vi "Release Queue.vi"(8 "error in (no error)":errorcluster, 11 "LVQueue Sink in":refnum<class "LVQueue Sink.lvclass">) -> (0 "error out":errorcluster, 3 "Remaining Elements":T1[](array[typedef]))   [LabVIEW 2018, in "MVA Framework.lvlib" / "LVQueue Sink.lvclass"]
uses:
  LVQueue Sink.lvclass
  Composed Log/Types/Log Level.ctl
  Composed Log/Composed Log.lvlib
  Composed Log/Types/Log Packet.ctl
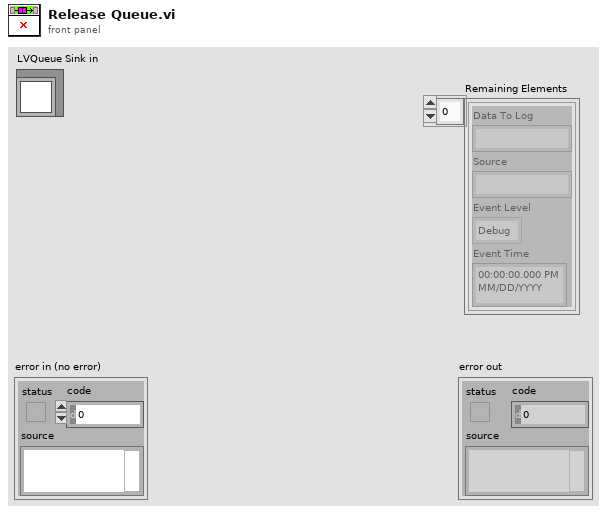
[diagram p1: front panel]
types:
  T1 = typedef "MVA Framework.lvlib/Composed Log.lvlib/Log Packet.ctl" = cluster{"Data To Log":string, "Source":string, "Event Level":T2, "Event Time":timestamp}
  T2 = typedef "MVA Framework.lvlib/Composed Log.lvlib/Log Level.ctl" = enum16{"Debug", "Info", "Warning", "Error", "Critical"}
  T3 = typedef "Composed Log.lvlib/Application Logger.lvclass/Log Packet.ctl" = cluster{"Data To Log":string, "Source":string, "Event Level":T4, "Event Time":timestamp}
  T4 = typedef "Composed Log.lvlib/Log Sink.lvclass/Log Level.ctl" = enum16{"Debug", "Info", "Warning", "Error", "Critical"}
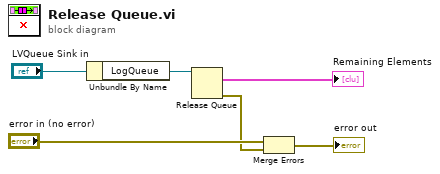
[diagram p0: block diagram]
diagram:
  n1 = Unbundle By Name("LVQueue Sink in") -> ("LogQueue"=w6:refnum<queue>)
  n2 = Release Queue(queue=w6) -> (remaining elements=→"Remaining Elements":T3[], error out=w3:errorcluster)  [unwired: 2 in, 1 out]
  n3 = Merge Errors("error in (no error)", w3) -> (→"error out":errorcluster)
